vi "Begin.vi"() -> (0 "error out":errorcluster)   [LabVIEW 2013]
doc: "Called before other user functions, this VI is expected to open initial I/O refnums, load in file data, and do all program initialization. Notice that the <B>error out</B> terminal is simply used for data flow. Wiring it to other structures or subVIs ensures that this VI runs first."
uses:
  <vilib>/Rock Robotics/WPI/RobotDrive/WPI_RobotDriveOpen2MotorWithJaguar.vi
  <vilib>/Rock Robotics/SystemInterfaces/DIO/FPGA_DIOPWMChannel.ctl
  <vilib>/Rock Robotics/WPI/SafetyOutput/WPI_SafetyOutputConfigMenu.ctl
  Robot Global Data.vi
  <vilib>/Rock Robotics/WPI/DriverStation/WPI_DriverStationRobotMode2.ctl
  <vilib>/Rock Robotics/WPI/Joystick/WPI_JoystickDeviceEnum.ctl
  <vilib>/Rock Robotics/WPI/MotorControl/WPI_MotorControlOpen Jaguar.vi
  <vilib>/Rock Robotics/SystemInterfaces/Typedef/FPGA_TypedefDigitalModule.ctl
  <vilib>/Rock Robotics/SystemInterfaces/DIO/FPGA_DIOChannel.ctl
  <vilib>/Rock Robotics/SystemInterfaces/DIO/FPGA_DIORelayChannel.ctl
panel:
  out "error out 2":errorcluster
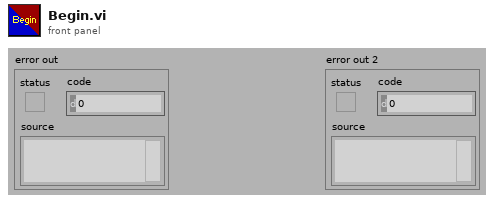
[diagram p1: front panel]
types:
  T1 = typedef "FPGA_TypedefDigitalModule.ctl" = enum16{"Digital Module 1", "Digital Module 2"}
  T2 = typedef "FPGA_DIORelayChannel.ctl" = enum8{"Relay 1", "Relay 2", "Relay 3", "Relay 4", "Relay 5", "Relay 6", "Relay 7", "Relay 8", "Invalid"}
  T3 = typedef "FPGA_DIOChannel.ctl" = enum8{"DIO 1", "DIO 2", "DIO 3", "DIO 4", "DIO 5", "DIO 6", "DIO 7", "DIO 8", "DIO 9", "DIO 10", "DIO 11", "DIO 12", "DIO 13", "DIO 14", "Invalid"}
  T4 = typedef "FPGA_DIOPWMChannel.ctl" = enum8{"PWM 1", "PWM 2", "PWM 3", "PWM 4", "PWM 5", "PWM 6", "PWM 7", "PWM 8", "PWM 9", "PWM 10", "Invalid"}
  T5 = typedef "WPI_JoystickDeviceEnum.ctl" = enum16{"USB 1", "USB 2", "USB 3", "USB 4", "Kinect 1", "Kinect 2"}
  T6 = typedef "WPI_DriverStationRobotMode2.ctl" = enum16{"Autonomous Disabled", "Autonomous Enabled", "Teleop Disabled", "Teleop Enabled", "Timeout", "Finish", "Test Disabled", "Test Enabled"}
  T7 = typedef "WPI_SafetyOutputConfigMenu.ctl" = enum16{"Enable", "Disable"}
  T8 = typedef "WPI_JoystickDevRef.ctl" = cluster{"Device":T5}
  T9 = typedef "WPI_RobotDriveDevRef.ctl" = cluster{"DevStatus":errorcluster, "Motors[]":T10[], "Square Inputs":bool, "Max Output":dbl, "Isochronous":bool}
  T10 = typedef "WPI_MotorControlDeviceRef.ctl" = cluster{"DeviceStatus":errorcluster, "Type":enum16{"PWM", "CAN"}, "PWM":cluster{"Digital Module":T1, "PWM Channel":T4, "DeadBand":T11}, "CAN":cluster{"Device Number":u8, "Control Mode":T12, "Semaphore":T13, "Max Vout":dbl}, "Invert":bool, "TransformRef":T14, "InvTransformRef":T14}
  T11 = typedef "WPI_PWMDeadband.ctl" = cluster{"Name":string, "maxPositivePwm":i32, "minPositivePwm":i32, "centerPwm":i32, "maxNegativePwm":i32, "minNegativePwm":i32, "angularRange":u16}
  T12 = typedef "WPI_CANJaguar_ControlMode.ctl" = enum8{"Percent VBus", "Current", "Speed", "Position", "Voltage"}
  T13 = typedef "Semaphore RefNum" = refnum<k1>
  T14 = typedef "WPI_PWMTransform_ConPane.ctl" = refnum<vi>
  T15 = typedef "WPI_CompressorDevRef.ctl" = cluster{"DevStatus":errorcluster, "DigitalInputDevRef":T16, "RelayDevRef":T17}
  T16 = typedef "WPI_DigitalInputDevRef.ctl" = cluster{"DevStatus":errorcluster, "DIO Channel":T3, "Digital Module":T1}
  T17 = typedef "WPI_RelayDevRef.ctl" = cluster{"DevStatus":errorcluster, "Relay Channel":T2, "Digital Module":T1, "Relay Direction":T18}
  T18 = typedef "WPI_RelayDirection.ctl" = enum16{"Both directions", "Forward only", "Reverse only"}
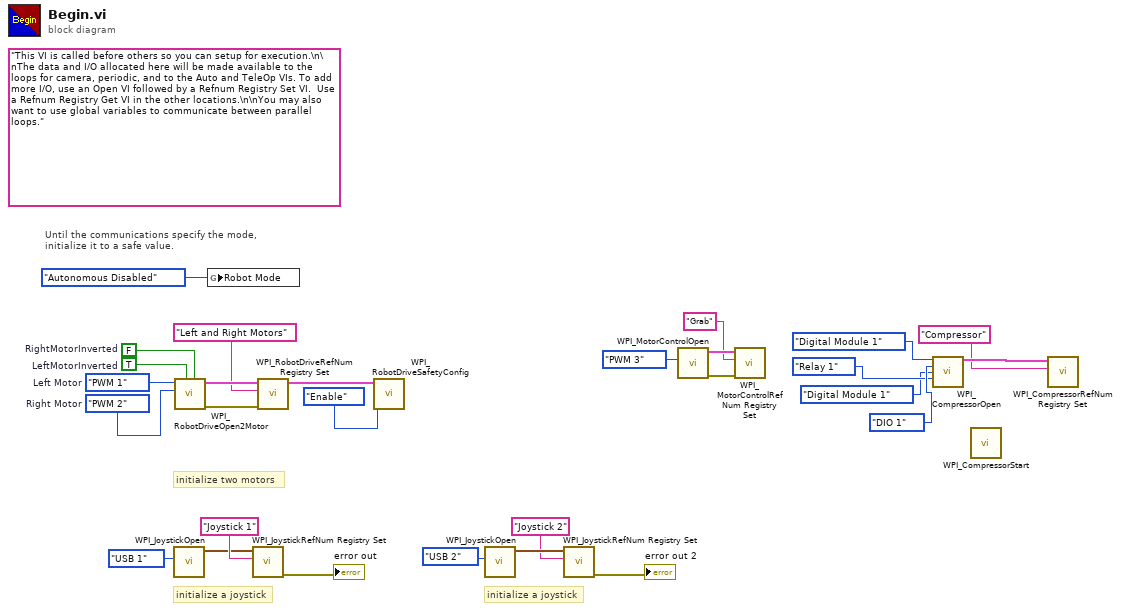
[diagram p0: block diagram]
diagram:
  (unwired) "This VI is called before others so you can setup for execution.\n\nThe data and I/O allocated here will be made available to the loops for camera, periodic, and to the Auto and TeleOp VIs. To add more I/O, use an Open VI followed by a Refnum Registry Set VI.  Use a Refnum Registry Get VI in the other locations.\n\nYou may also want to use global variables to communicate between parallel loops."
  w22 = FPGA_DIOPWMChannel."PWM 2"  # Right Motor
  w23 = FPGA_DIOPWMChannel."PWM 1"  # Left Motor
  w27 = TRUE  # LeftMotorInverted
  w28 = FALSE  # RightMotorInverted
  # "initialize a joystick"
  # "initialize a joystick"
  # "Until the communications specify the mode,\ninitialize it to a safe value."
  # "initialize two motors"
  n1 = call <vilib>:"WPI_JoystickOpen.vi"("JoystickDevice"=WPI_JoystickDeviceEnum."USB 1") -> ("JoystickDevRef"=w17:T8)  [unwired: 10 in]
  n2 = call-poly <vilib>:"WPI_RobotDriveOpen2Motor.vi"("Right Motor Inverted"=w28, "Left Motor Inverted"=w27, "Right Motor"=w22, "Left Motor"=w23) -> ("error out"=w24:errorcluster, "RobotDriveDevRef"=w26:T9)  [unwired: 1 in, 5 out]
  n3 = global write "Robot Global Data.vi" "Robot Mode"(WPI_DriverStationRobotMode2."Autonomous Disabled" ("Robot Mode")) -> ()
  n4 = call <vilib>:"WPI_JoystickRefNum Registry Set.vi"("refnum name"="Joystick 1", "JoystickDevRef"=w17) -> ("error out"=→"error out":errorcluster)  [unwired: 8 in, 1 out]
  n5 = call <vilib>:"WPI_RobotDriveRefNum Registry Set.vi"("error in (no error)"=w24, "refnum name"="Left and Right Motors", "RobotDriveDevRef"=w26) -> ("RobotDriveDevRef"=w21:T9)  [unwired: 8 out]
  n6 = call <vilib>:"WPI_RobotDriveSafetyConfig.vi"("mode"=WPI_SafetyOutputConfigMenu."Enable", "RobotDriveDevRef"=w21) -> ()  [unwired: 8 in, 2 out]
  n7 = call <vilib>:"WPI_JoystickOpen.vi"("JoystickDevice"=WPI_JoystickDeviceEnum."USB 2") -> ("JoystickDevRef"=w12:T8)  [unwired: 10 in]
  n8 = call <vilib>:"WPI_JoystickRefNum Registry Set.vi"("refnum name"="Joystick 2", "JoystickDevRef"=w12) -> ("error out"=→"error out 2":errorcluster)  [unwired: 8 in, 1 out]
  n9 = call-poly <vilib>:"WPI_MotorControlOpen.vi"("PWM Channel"=FPGA_DIOPWMChannel."PWM 3") -> ("error out"=w10:errorcluster, "MotorControlDeviceRef"=w9:T10)  [unwired: 9 in]
  n10 = call <vilib>:"WPI_MotorControlRefNum Registry Set.vi"("error in (no error)"=w10, "refnum name"="Grab", "MotorControlDevRef"=w9) -> ()  [unwired: 7 in, 2 out]
  n11 = call <vilib>:"WPI_CompressorOpen.vi"("Pressure Switch Digital Module (Module 1)"=FPGA_TypedefDigitalModule."Digital Module 1", "Pressure Switch DIO Channel"=FPGA_DIOChannel."DIO 1", "Relay Digital Module (Module 1)"=FPGA_TypedefDigitalModule."Digital Module 1", "Relay Channel"=FPGA_DIORelayChannel."Relay 1") -> ("CompressorDevRef"=w6:T15)  [unwired: 10 in, 1 out]
  n12 = call <vilib>:"WPI_CompressorStart.vi"() -> ()  [unwired: 10 in, 2 out]
  n13 = call <vilib>:"WPI_CompressorRefNum Registry Set.vi"("refnum name"="Compressor", "CompressorDevRef"=w6) -> ()  [unwired: 8 in, 2 out]
